vi "call rust.vi"   [LabVIEW 2019]
uses:
  rust/target/debug/rust_outputs.dll
types:
  T1 = cluster{"t0":timestamp, "dt":dbl, "values":dbl[]}
  T2 = cluster{"f0":dbl, "df":dbl, "values":dbl[], "centre_time":timestamp}[]
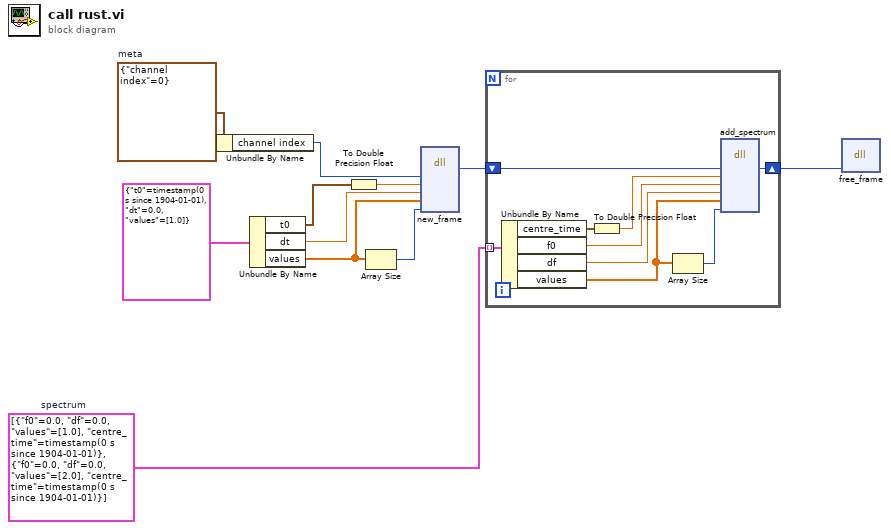
[diagram p0: block diagram]
diagram:
  w1 = T2 [{"f0"=0.0, "df"=0.0, "values"=[1.0], "centre_time"=timestamp(0 s since 1904-01-01)}, {"f0"=0.0, "df"=0.0, "values"=[2.0], "centre_time"=timestamp(0 s since 1904-01-01)}]  # spectrum
  w11 = cluster{"channel index":i32} {"channel index"=0}  # meta
  n1 = Unbundle By Name(w11) -> ("channel index"=w10:i32)
  n2 = Unbundle By Name(T1 {"t0"=timestamp(0 s since 1904-01-01), "dt"=0.0, "values"=[1.0]} ("spectrum")) -> ("t0"=w6:timestamp, "dt"=w8:dbl, "values"=w5:dbl[])
  n3 = To Double Precision Float(number=w6) -> (double precision float=w7:dbl)
  n4 = Array Size(array=w5) -> (size(s)=w4:i32)
  n5 = dll-call lib="C:/Users/james.WIRESMITH/Documents/Rust-From-LabVIEW/rust/target/debug/rust_outputs.dll" fn="new_frame"("channel_idx"=w10, "t0_timestamp"=w7, "dt"=w8, "waveform_values"=w5, "waveform_size"=w4) -> ("return type"=w3:u64)  [unwired: 8 in, 2 out]
  n6 = for {
    shift-right: [w19] -> w2
    shift-left: w3 -> [w20]
    tunnel: w1 -> [w18] mode=indexing
    n7 = Unbundle By Name(w18) -> ("centre_time"=w17:timestamp, "f0"=w15:dbl, "df"=w14:dbl, "values"=w13:dbl[])
    n8 = To Double Precision Float(number=w17) -> (double precision float=w16:dbl)
    n9 = Array Size(array=w13) -> (size(s)=w12:i32)
    n10 = dll-call lib="C:/Users/james.WIRESMITH/Documents/Rust-From-LabVIEW/rust/target/debug/rust_outputs.dll" fn="add_spectrum"("frame_ptr"=w20, "timestamp"=w16, "f0"=w15, "df"=w14, "values"=w13, "size"=w12) -> ("frame_ptr"=w19:u64)  [unwired: 9 in, 2 out]
  }
  n11 = dll-call lib="C:/Users/james.WIRESMITH/Documents/Rust-From-LabVIEW/rust/target/debug/rust_outputs.dll" fn="free_frame"("frame_ptr"=w2) -> ()  [unwired: 5 in, 2 out]
